vi "Osciloscopio.vi"() -> ()   [LabVIEW 2015]
uses:
  <vilib>/measure/NI_MABase.lvlib
panel:
  in  "stop":bool
  in  "Amplitud":dbl(knob) scale=0.0..20.0
  in  "Frecuencia":dbl(knob) scale=0.0..20.0
  out "Waveform Graph":waveform(dbl)(graph)
  out "Waveform Chart":waveform(dbl)(graph)
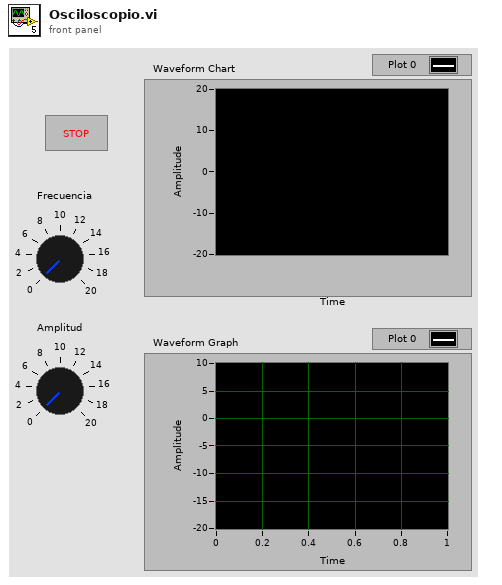
[diagram p1: front panel]
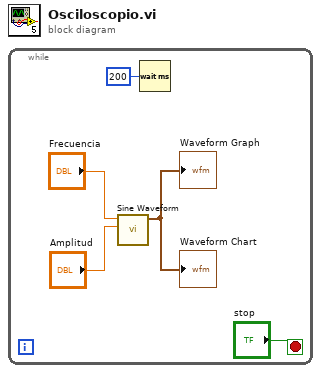
[diagram p0: block diagram]
diagram:
  n1 = while {
    stop <- "stop" stop-if-true
    n2 = call <vilib>:"Sine Waveform.vi"("amplitude"="Amplitud", "frequency"="Frecuencia") -> ("signal out"=→"Waveform Chart" →"Waveform Graph":waveform(dbl))  [unwired: 8 in, 1 out]
    n3 = Wait (ms)(milliseconds to wait=u32 200) -> ()  [unwired: 1 out]
  }
